vi "QuitOnLastWindowClosed-Get.vi"(8 "error in (no error)":errorcluster, 11 "Engine in":refnum<class "Engine.lvclass">) -> (0 "error out":errorcluster, 2 "Quit On Last Window Closed":bool, 3 "Engine out":refnum<class "Engine.lvclass">)   [LabVIEW 2024, in "GLF.lvlib" / "Engine.lvclass"]
uses:
  Engine.lvclass
  Engine.lvclass/Engine.ctl
  a1934f40-8091-4efc-9cde-54247e41822d.vi
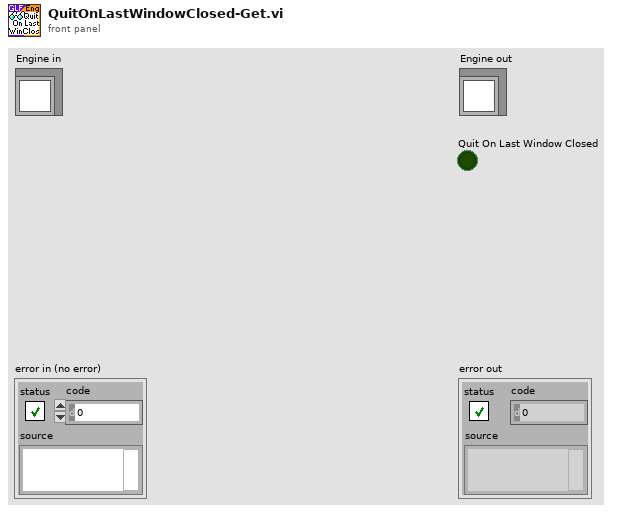
[diagram p1: front panel]
types:
  T1 = typedef "GLF.lvlib/Engine.lvclass/DVR--cluster.ctl" = cluster{"CMD Queue":T2, "Config":T3, "Ctxt":T5, "Metrics":T6}
  T2 = typedef "GLF.lvlib/Engine.lvclass/Command--queue.ctl" = refnum<queue>
  T3 = typedef "GLF.lvlib/Engine.lvclass/Config--cluster.ctl" = cluster{"Quit On Last Window Closed":bool, "VSync":T4, "FPS Target":dbl}
  T4 = typedef "GLF.lvlib/Engine.lvclass/VSync--enum.ctl" = enum16{"Disabled", "Enabled", "Adaptative"}
  T5 = typedef "GLF.lvlib/Engine.lvclass/Context--cluster.ctl" = cluster{"Ticks Begin":u64, "VSync Enabled":bool}
  T6 = typedef "GLF.lvlib/Engine.lvclass/Metrics--cluster.ctl" = cluster{"Uptime [ms]":u64, "Loop Time [ms]":u64}
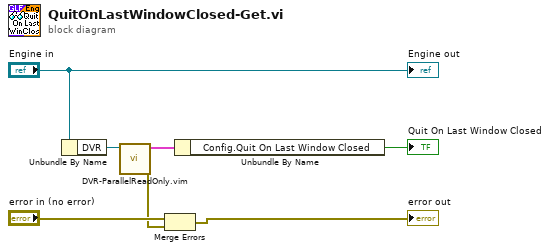
[diagram p0: block diagram]
diagram:
  n1 = Unbundle By Name("Engine in") -> ("DVR"=w4:refnum<data-value>)
  n2 = call "DVR-ParallelReadOnly.vim"("DVR"=w4) -> ("Error Out"=w2:errorcluster, "Data"=w3:T1)  [unwired: 9 in]
  n3 = Merge Errors("error in (no error)", w2) -> (→"error out":errorcluster)
  n4 = Unbundle By Name(w3) -> ("Config.Quit On Last Window Closed"=→"Quit On Last Window Closed":bool)
  "Engine out" <- "Engine in"
